vi "Cluster AutoSizing - Arrange Veritcally.vi"(6 "Variant in":variant, 7 "Shift Pressed?":bool, 8 "error in (no error)":errorcluster, 10 "QD Combo Box Ref":refnum<vi>, 11 "QD Launch VI Ref":refnum<vi>) -> (0 "error out":errorcluster, 4 "Variant out":variant)   [LabVIEW 2017, in "Cluster AutoSizing.lvlib"]
doc: "Sets the auto-sizing mode of the selected clusters to Arrange Vertically. Hold Shift to apply it to the clusters contained in them as well."
uses:
  Cluster AutoSizing.lvlib
panel:
  in  "Undo Name":string="Cluster autosizing"
  # "Do not change the connector pane of this VI.\n\nSee the block diagram for directions on how to use this template."
  # "Specify the name of the Undo transaction"
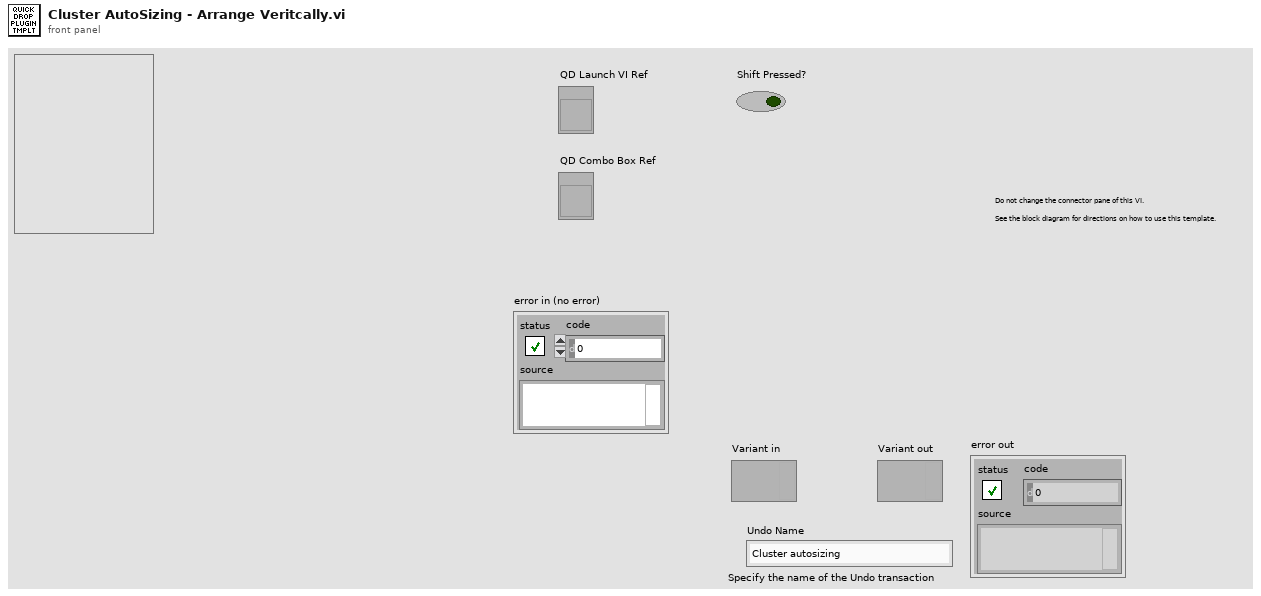
[diagram p1: front panel]
types:
  T1 = enum16{"None", "Size to Fit", "Arrange Horizontally", "Arrange Veritcally"}
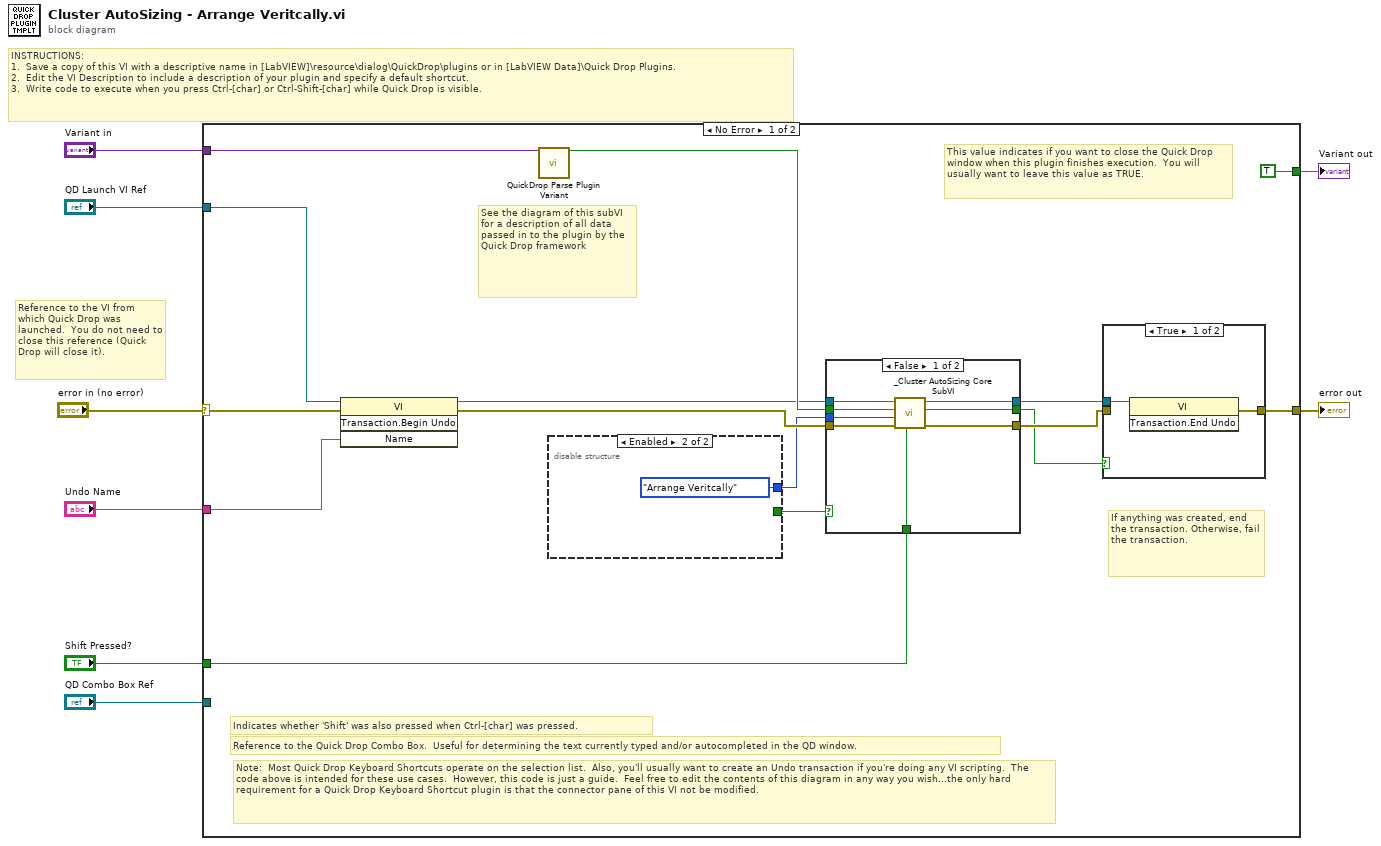
[diagram p0: block diagram]
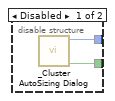
[diagram p2: hidden frame]
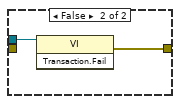
[diagram p4: hidden frame]
diagram:
  # "Reference to the VI from which Quick Drop was launched.  You do not need to close this reference (Quick Drop will close it)."
  # "INSTRUCTIONS:\n1.  Save a copy of this VI with a descriptive name in [LabVIEW]\\resource\\dialog\\QuickDrop\\plugins or in [LabVIEW Data]\\Quick Drop Plugins.\n2.  Edit the VI Description to include a description of your plugin and specify a default shortcut. \n3.  Write code to execute when you press Ctrl-[char] or Ctrl-Shift-[char] while Quick Drop is visible."
  n1 = case shown="No Error" "error in (no error)" {
    selector: "error in (no error)" -> [w22 w41]
    tunnel: [w16 w41] -> w8
    tunnel: "QD Launch VI Ref" -> [w21 _]
    tunnel: "Shift Pressed?" -> [w9 _]
    tunnel: "QD Combo Box Ref" -> [_ _]
    tunnel: "Variant in" -> [w23 _]
    tunnel: "Undo Name" -> [w20 _]
    tunnel: [TRUE _] -> w2
    frame No Error {
      # "Note:  Most Quick Drop Keyboard Shortcuts operate on the selection list.  Also, you'll usually want to create an Undo transaction if you're doing any VI scripting.  The code above is intended for these use cases.  However, this code is just a guide.  Feel free to edit the contents of this diagram in any way you wish...the only hard requirement for a Quick Drop Keyboard Shortcut plugin is that the connector pane of this VI not be modified."
      # "If anything was created, end the transaction. Otherwise, fail the transaction."
      # "This value indicates if you want to close the Quick Drop window when this plugin finishes execution.  You will usually want to leave this value as TRUE."
      # "See the diagram of this subVI for a description of all data passed in to the plugin by the Quick Drop framework"
      # "Reference to the Quick Drop Combo Box.  Useful for determining the text currently typed and/or autocompleted in the QD window."
      # "Indicates whether 'Shift' was also pressed when Ctrl-[char] was pressed."
      n2 = invoke class="VI" method="Transaction.Begin Undo"(reference=w21, error in=w22, "Name"=w20) -> (reference out=w12:refnum<vi>, error out=w17:errorcluster)  [unwired: 1 in, 2 out]
      n3 = call <vilib>:"QuickDrop Parse Plugin Variant.vi"("QDKS Variant in"=w23) -> ("QD Launch VI Panel?"=w18:bool)  [unwired: 12 in, 2 out]
      n4 = disable-structure shown="Enabled" {
        disable-tunnel: [w25 T1."Arrange Veritcally" ("type")] -> w14
        disable-tunnel: [w24 _] -> w10
        frame Disabled {
          n5 = call "_Cluster AutoSizing Dialog.vi"() -> ("cancelled?"=w24:bool, "type"=w25:T1)  [unwired: 9 in, 1 out]
        }
        frame Enabled {
        }
      }
      n6 = case shown="False" w10 {
        tunnel: w18 -> [w34 _]
        tunnel: w17 -> [w33 w35]
        tunnel: [w32 w35] -> w15
        tunnel: w14 -> [w31 _]
        tunnel: [w30 _] -> w13
        tunnel: w12 -> [w29 w36]
        tunnel: [w28 w36] -> w11
        tunnel: w9 -> [w27 _]
        frame False {
          n7 = call "_Cluster AutoSizing Core SubVI.vi"("recursive"=w27, "error in (no error)"=w33, "type"=w31, "QD Launch VI Panel?"=w34, "VI in"=w29) -> ("error out"=w32:errorcluster, "Changed?"=w30:bool, "VI out"=w28:refnum<vi>)  [unwired: 4 in]
        }
        frame True {
        }
      }
      n8 = case shown="True" w13 {
        tunnel: w11 -> [w37 w39]
        tunnel: [w38 w40] -> w16
        tunnel: w15 -> [_ _]
        frame True {
          n9 = invoke class="VI" method="Transaction.End Undo"(reference=w37) -> (error out=w38:errorcluster)  [unwired: 2 in, 2 out]
        }
        frame False {
          n10 = invoke class="VI" method="Transaction.Fail"(reference=w39) -> (error out=w40:errorcluster)  [unwired: 2 in, 2 out]
        }
      }
    }
    frame Error {
    }
  }
  "error out" <- w8
  "Variant out" <- w2
